vi "__Test Load XML Report Plugin.vi"(8 "error in (no error)":errorcluster, 11 "Plugin Loader Tests in":refnum<class "Plugin Loader Tests.lvclass">) -> (0 "error out":errorcluster, 3 "Plugin Loader Tests out":refnum<class "Plugin Loader Tests.lvclass">)   [LabVIEW 2020, in "Plugin Loader Tests.lvclass"]
uses:
  Plugin Loader Tests.lvclass
  Plugin Loader Tests.lvclass/Plugin Loader Tests.ctl
  249b0d5c-641c-4737-bb7b-a27b44f239ac.vi
  source/User Interface/Plugin Loader/Plugin Loader.lvclass
  source/Plugins/XML Report/XML Report.lvclass
  source/Framework/Plugin/Plugin.lvclass
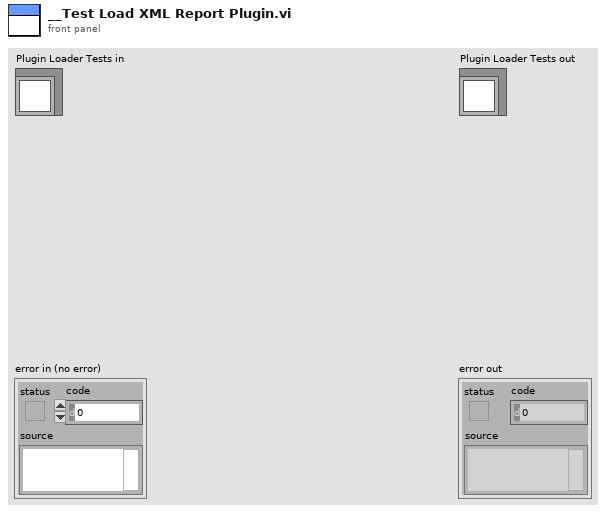
[diagram p1: front panel]
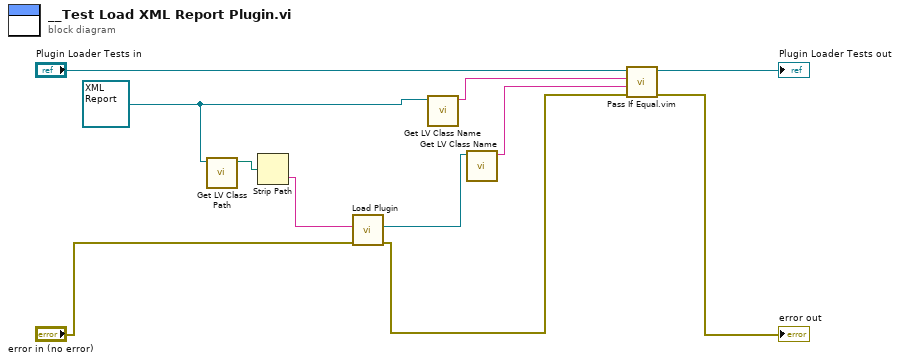
[diagram p0: block diagram]
diagram:
  w2 = refnum<class "XML Report.lvclass"> refnum ("Reports.lvlib:XML Report.lvclass")
  n1 = call <vilib>:"Get LV Class Path.vi"("object"=w2) -> ("class path"=w3:path)  [unwired: 9 in, 1 out]
  n2 = Strip Path(path=w3) -> (name=w1:string)  [unwired: 1 out]
  n3 = call "Load Plugin.vi"("error in (no error)"="error in (no error)", "Plugin"=w1) -> ("error out"=w7:errorcluster, "Plugin"=w6:refnum<class "Plugin.lvclass">)  [unwired: 8 in]
  n4 = call <vilib>:"Get LV Class Name.vi"("object"=w2) -> ("class name"=w4:string)  [unwired: 9 in, 1 out]
  n5 = call <vilib>:"Get LV Class Name.vi"("object"=w6) -> ("class name"=w5:string)  [unwired: 9 in, 1 out]
  n6 = call "Pass If Equal.vim"("error in (no error)"=w7, "Actual"=w5, "Expected"=w4, "LUnit Test Case In"="Plugin Loader Tests in") -> ("error out"=→"error out":errorcluster, "LUnit Test Case Out"=→"Plugin Loader Tests out":refnum<class "Plugin Loader Tests.lvclass">)  [unwired: 6 in]
